vi "Set Data on Point.vi"(0 "eye scan point iterator":refnum<class "niHighSpeedSerial Rectangular Eye Scan Point Iterator v1 Host.lvclass">, 5 "bit error ratio":dbl, 7 "sample count":u64, 9 "error count":u64, 11 "error in":errorcluster) -> (4 "eye scan point iterator out":refnum<class "niHighSpeedSerial Rectangular Eye Scan Point Iterator v1 Host.lvclass">, 15 "error out":errorcluster)   [LabVIEW 2014, in "niHighSpeedSerial Rectangular Eye Scan Point Iterator v1 Host.lvclass"]
doc: "Sets the specified data on the active point.\n\n<B>Input Parameters</B>\n\n<B>eye scan point iterator</B> is the incoming wire for the Eye Scan Point Iterator class object\n\n<B>bit error rate</B> is the calculated statistical bit error rate based on the number of error counts and sample counts received.\n\n<B>sample count</B> is the number of samples that have been measured on this point.\n\n<B>error count</B> is the number of errors that have been measured on this point.\n\n<B>error in</B> describes error conditions that occur before this node runs. This input provides standard 'error in' functionality.\n\n<B>Output Parameters</B>\n\n<B>eye scan point iterator out</B> is the outgoing wire for the Eye Scan Point Iterator class object\n\n<B>error out</B> contains error information. This output provides standard 'error out' functionality."
uses:
  <instrlib>/niHighSpeedSerial/Eye Scan/v1/Host/Impl/Rect Iter/niHighSpeedSerial Rectangular Eye Scan Point Iterator v1 Host.lvclass
  <instrlib>/niHighSpeedSerial/Eye Scan/v1/Host/Impl/Rect Iter/niHighSpeedSerial Rectangular Eye Scan Point Iterator v1 Host.lvclass/niHighSpeedSerial Rectangular Eye Scan Point Iterator v1 Host.ctl
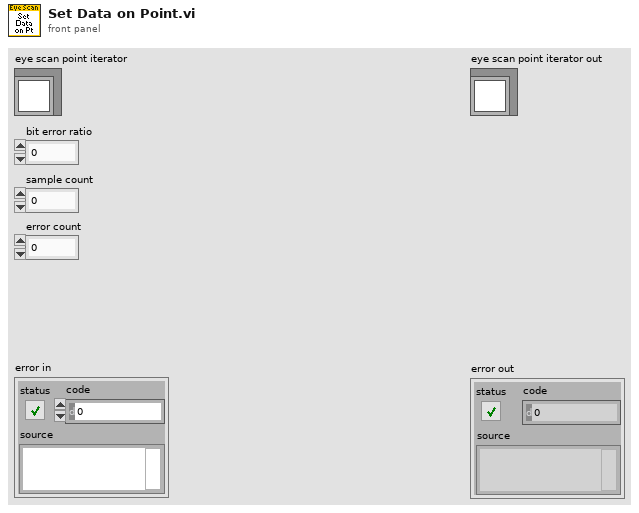
[diagram p1: front panel]
types:
  T1 = typedef "niHighSpeedSerial Eye Scan Common v1 Host.lvlib/Point.ctl" = cluster{"point offsets":T2, "sample count":u64, "error count":u64, "bit error ratio":dbl}
  T2 = typedef "niHighSpeedSerial Eye Scan Common v1 Host.lvlib/Point Offsets.ctl" = cluster{"horizontal offset":i16, "vertical offset":i8}
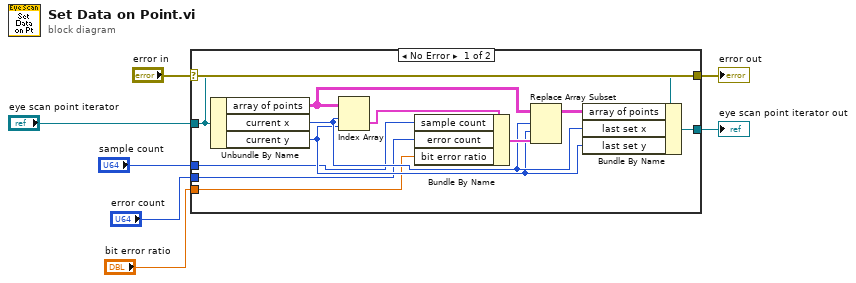
[diagram p0: block diagram]
diagram:
  n1 = case shown="No Error" "error in" {
    selector: "error in" -> [w19 w21]
    tunnel: [w19 w21] -> w6
    tunnel: "eye scan point iterator" -> [w14 w20]
    tunnel: [w13 w20] -> w4
    tunnel: "error count" -> [w10 _]
    tunnel: "sample count" -> [w9 _]
    tunnel: "bit error ratio" -> [w8 _]
    frame No Error {
      n2 = Unbundle By Name(w14) -> ("array of points"=w17:T1[][], "current x"=w12:i32, "current y"=w11:i32)
      n3 = Index Array(array=w17, index (row)=w12, index (col)=w11) -> (element=w18:T1)
      n4 = Bundle By Name(cluster=w18, "sample count"=w9, "error count"=w10, "bit error ratio"=w8) -> (w16:T1)
      n5 = Replace Array Subset(array=w17, new element=w16, index (row)=w12, index (col)=w11) -> (w15:T1[][])
      n6 = Bundle By Name(cluster=w14, "array of points"=w15, "last set x"=w12, "last set y"=w11) -> (w13:refnum<class "niHighSpeedSerial Rectangular Eye Scan Point Iterator v1 Host.lvclass">)
    }
    frame Error {
    }
  }
  "error out" <- w6
  "eye scan point iterator out" <- w4
